vi "Test Internet.vi"(8 "error in (no error)":errorcluster) -> (0 "Available":bool, 1 "error out":errorcluster)   [LabVIEW 2016]
panel:
  out "Result":string
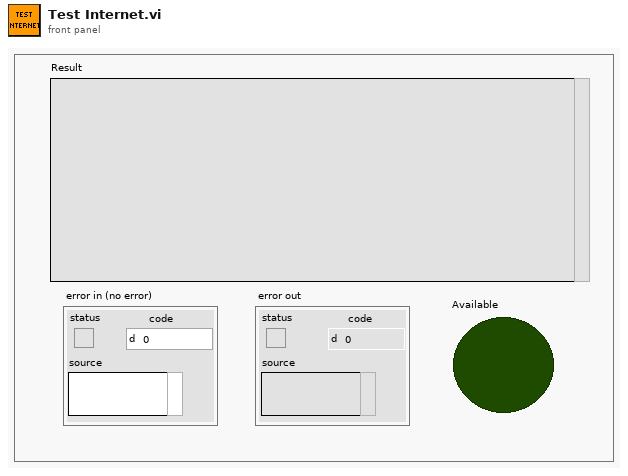
[diagram p1: front panel]
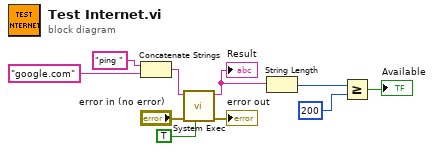
[diagram p0: block diagram]
diagram:
  n1 = Concatenate Strings("ping " ("command line"), "google.com" ("PC Name or IP Address")) -> (w10:string)
  n2 = call <vilib>:"System Exec.vi"("run minimized? (F)"=TRUE, "error in (no error)"="error in (no error)", "command line"=w10) -> ("error out"=→"error out":errorcluster, "standard output"=w4:string)  [unwired: 3 in, 4 out]
  "Result" <- w4
  n3 = String Length(string=w4) -> (length=w3:i32)
  n4 = Greater Or Equal?(x=w3, y=200) -> (x >= y?=→"Available":bool)
